vi "da TIPO a ID.vi"(11 "TIPO":string) -> (3 "ID":i32)   [LabVIEW 2019]
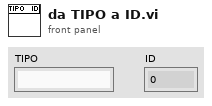
[diagram p1: front panel]
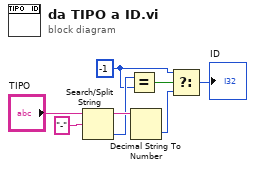
[diagram p0: block diagram]
diagram:
  w1 = -1 ("y")
  n1 = Search/Split String(string="TIPO", search string/char (-)="-") -> (substring before match=w8:string, offset of match=w5:i32)  [unwired: 1 in, 1 out]
  n2 = Equal?(x=w5, y=w1) -> (x = y?=w2:bool)
  n3 = Decimal String To Number(string=w8) -> (number=w4:i32)  [unwired: 2 in, 1 out]
  n4 = Select(t=w1, s=w2, f=w4) -> (s? t:f=→"ID":i32)
